vi "calibration method2.vi"(1 "function name":string="fit", 5 "Image IN":T1(plugin-control), 7 "initialize matrix":dbl[][](array[numeric]), 9 "module path":path, 11 "error in":errorcluster, 12 "snap number":i32) -> (8 "calibration matrix":dbl[][](array[numeric]), 15 "error out":errorcluster)   [LabVIEW 2019, in "Calibration Lib.lvlib"]
uses:
  Calibration Lib.lvlib
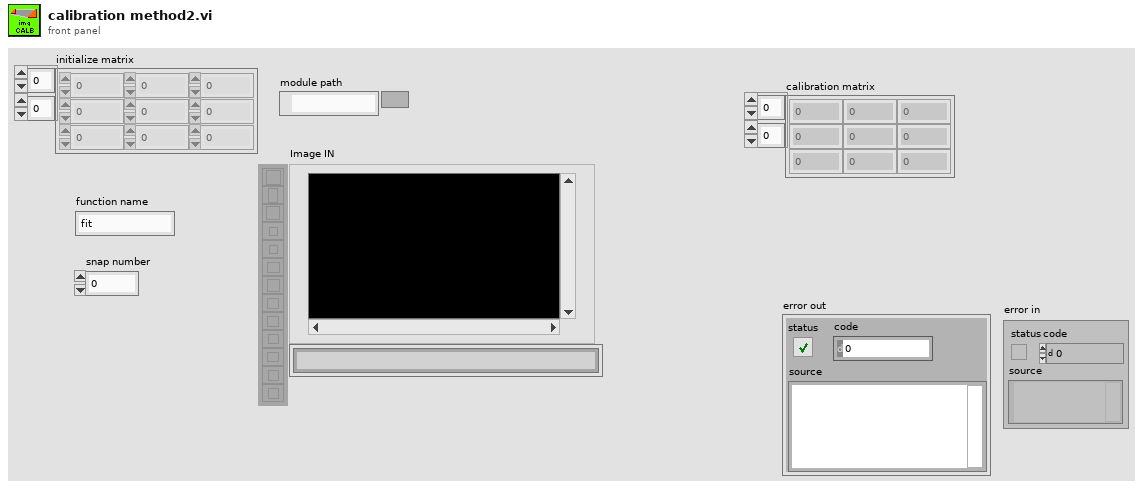
[diagram p1: front panel]
types:
  T1 = typedef "IMAQ Image.ctl" = refnum<image>
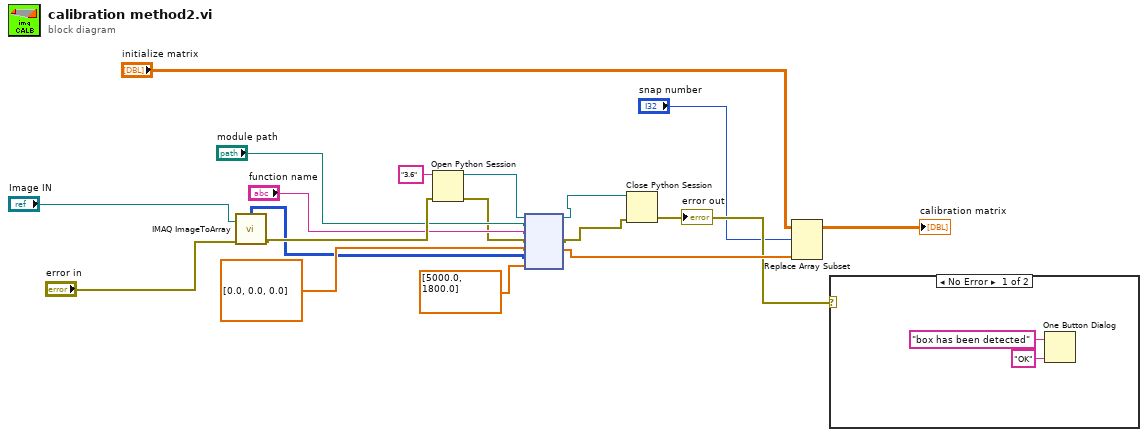
[diagram p0: block diagram]
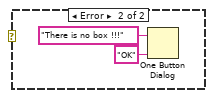
[diagram p2: hidden frame]
diagram:
  n1 = call "IMAQ ImageToArray"("error in (no error)"="error in", "Image"="Image IN") -> ("error out"=w13:errorcluster, "Image Pixels (U8)"=w7:u8[][])  [unwired: 2 in, 3 out]
  n2 = Open Python Session(python version="3.6" ("Python version"), 3:w13) -> (session out=w12:refnum<k35>, error out=w9:errorcluster)  [unwired: 1 in]
  n3 = node(w12, "module path", "function name", w9, dbl[] [0.0, 0.0, 0.0], w7, dbl[] [5000.0, 1800.0]) -> (w5:refnum<k35>, w4:errorcluster, w3:dbl[])  [unwired: 2 in, 2 out]
  n4 = Close Python Session(session in=w5, error in=w4) -> (11:w2:errorcluster)
  "error out" <- w2
  n5 = Replace Array Subset(array="initialize matrix", new element=w3, index (row)="snap number") -> (→"calibration matrix":dbl[][])  [unwired: 1 in]
  n6 = case shown="No Error" w2 {
    frame No Error {
      n7 = One Button Dialog(message="box has been detected", button name ("OK")="OK") -> ()  [unwired: 1 out]
    }
    frame Error {
      n8 = One Button Dialog(message="There is no box !!!", button name ("OK")="OK") -> ()  [unwired: 1 out]
    }
  }
